vi "Get Modules.vi"(11 "Module list in":string[](array[string])) -> (1 "Destination Map":map{string, string[]}(c390), 2 "Module Map":map{string, refnum<class "Module.lvclass">}(c390), 3 "Conjunctions out":string[](array[string]))   [LabVIEW 2021]
uses:
  Day 20/Module/Module.lvclass
  Day 20/Flipflop/Flipflop.lvclass
  C:/Projects/LabVIEWAdventOfCode2023/Day 20/Module/Module.lvclass
  Day 20/Conjunction/Conjunction.lvclass
  Day 20/Broadcaster/Broadcaster.lvclass
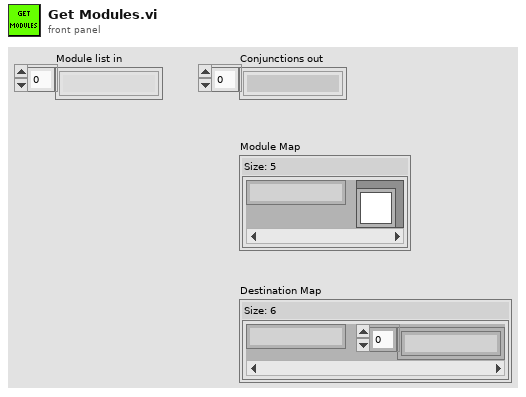
[diagram p1: front panel]
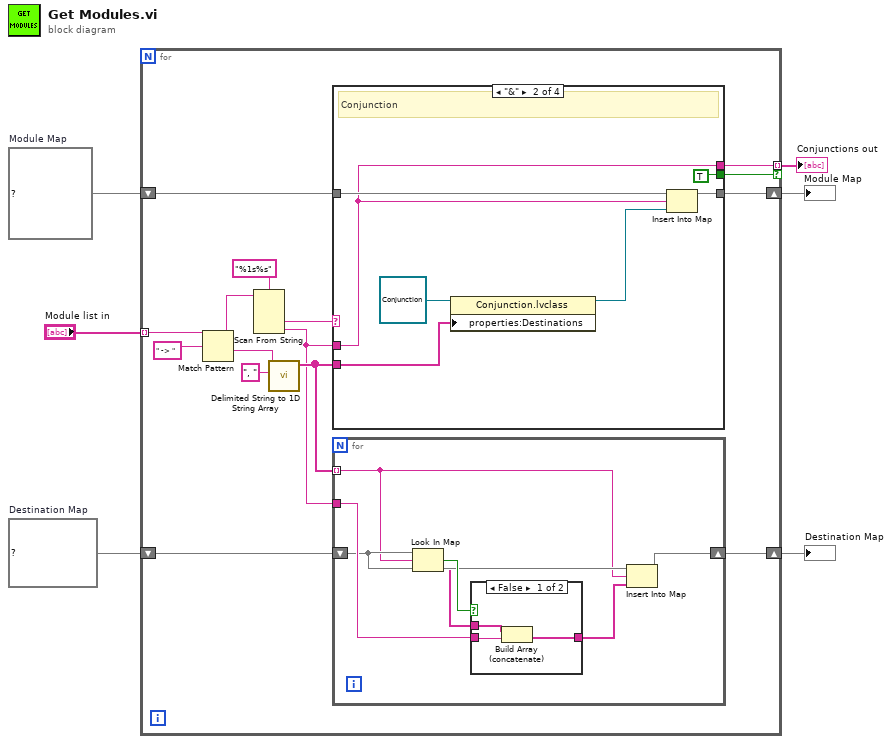
[diagram p0: block diagram]
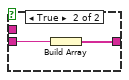
[diagram p2: hidden frame]
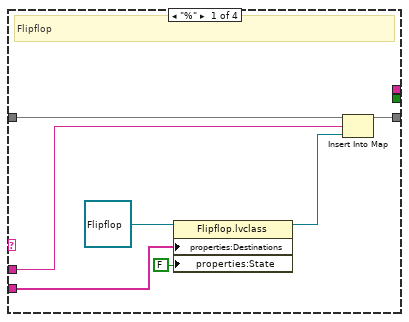
[diagram p3: hidden frame]
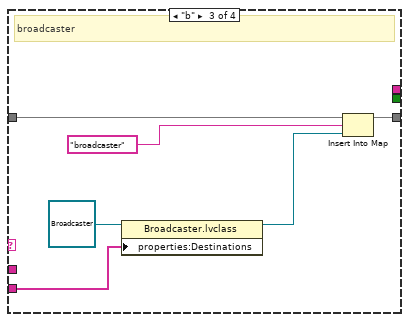
[diagram p4: hidden frame]
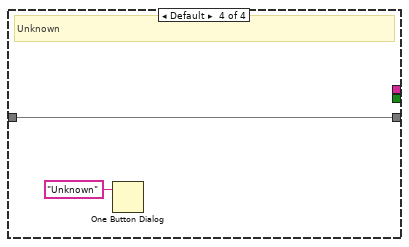
[diagram p5: hidden frame]
diagram:
  w3 = map{string, string[]} {}  # Destination Map
  w2 = map{string, refnum<class "Module.lvclass">} {}  # Module Map
  n1 = for {
    tunnel: "Module list in" -> [w21] mode=indexing
    shift-right: [w13] -> w5
    shift-left: w2 -> [w14]
    tunnel: [w12] -> w4 mode=indexing if=w7
    shift-right: [w8] -> w6
    shift-left: w3 -> [w9]
    n2 = Match Pattern(string=w21, regular expression=" -> ") -> (before substring=w17:string, after substring=w19:string)  [unwired: 1 in, 2 out]
    n3 = Scan From String(format string="%1s%s", input string=w17) -> (output 1=w15:string, output 2=w10:string)  [unwired: 4 in, 3 out]
    n4 = call <vilib>:"Delimited String to 1D String Array.vi"("delimiter"=", ", "delimited string"=w19) -> ("string array"=w11:string[])  [unwired: 9 in]
    n5 = case shown="\"&\"" w15 {
      tunnel: w10 -> [w38 w42 _ _]
      tunnel: w11 -> [w35 w45 w49 _]
      tunnel: w14 -> [w40 w47 w53 w55]
      tunnel: [w39 w46 w52 w55] -> w13
      tunnel: [_ w42 _ _] -> w12
      tunnel: [_ TRUE _ _] -> w7
      frame "%" {
        # "Flipflop"
        n6 = property class="Flipflop.lvclass"(reference=refnum<class "Flipflop.lvclass"> refnum ("Flipflop.lvclass"), "properties:Destinations"=w35, "properties:State"=FALSE) -> (reference out=w34:refnum<class "Flipflop.lvclass">)  [unwired: 1 in, 1 out]
        n7 = Insert Into Map(map in=w40, key=w38, value=w34) -> (map out=w39:map{string, refnum<class "Module.lvclass">})  [unwired: 2 out]
      }
      frame "&" {
        # "Conjunction"
        n8 = property class="Conjunction.lvclass"(reference=refnum<class "Conjunction.lvclass"> refnum ("Conjunction.lvclass"), "properties:Destinations"=w45) -> (reference out=w44:refnum<class "Conjunction.lvclass">)  [unwired: 1 in, 1 out]
        n9 = Insert Into Map(map in=w47, key=w42, value=w44) -> (map out=w46:map{string, refnum<class "Module.lvclass">})  [unwired: 2 out]
      }
      frame "b" {
        # "broadcaster"
        n10 = property class="Broadcaster.lvclass"(reference=refnum<class "Broadcaster.lvclass"> refnum ("Broadcaster.lvclass"), "properties:Destinations"=w49) -> (reference out=w48:refnum<class "Broadcaster.lvclass">)  [unwired: 1 in, 1 out]
        n11 = Insert Into Map(map in=w53, key="broadcaster", value=w48) -> (map out=w52:map{string, refnum<class "Module.lvclass">})  [unwired: 2 out]
      }
      frame Default {
        # "Unknown"
        n12 = One Button Dialog(message="Unknown") -> ()  [unwired: 1 in, 1 out]
      }
    }
    n13 = for {
      tunnel: w11 -> [w24] mode=indexing
      tunnel: w10 -> [w27]
      shift-right: [w25] -> w8
      shift-left: w9 -> [w26]
      n14 = Look In Map(map=w26, key=w24) -> (key not found?=w28:bool, value=w22:string[])  [unwired: 1 in]
      n15 = case shown="False" w28 {
        tunnel: w27 -> [w31 w33]
        tunnel: [w29 w32] -> w23
        tunnel: w22 -> [w30 _]
        frame False {
          n16 = Build Array (concatenate)(w30, w31) -> (w29:string[])
        }
        frame True {
          n17 = Build Array(w33) -> (w32:string[])
        }
      }
      n18 = Insert Into Map(map in=w26, key=w24, value=w23) -> (map out=w25:map{string, string[]})  [unwired: 2 out]
    }
  }
  "Destination Map" <- w6
  "Module Map" <- w5
  "Conjunctions out" <- w4
